vi "主画面.vi"() -> ()   [LabVIEW 2016]
panel:
  out "连接的字符串":string
  in  "邮件按钮":bool
  in  "配置信息":T1={"address"="27.154.58.30", "username"="admin", "password"="std23506", "filename"="一体化微型水质监测站.exe", "localpath"="C:\\Users\\Administrator\\Desktop\\ftp接收文件\\一体化微型水质监测站.exe"}
  out "字符串":string
  in  "启用":bool
  in  "选择站点":bool[](array[boolean])
  out "information":T2(array[cluster])
  in  "多列列表框":i32[](listbox)
  out "子字符串;substring":string
  in  "Port":u16=10000
  in  "empty":refnum<k5>[](array[refnum])
  out "# of Connections":i32
  in  "stop":bool
  in  "listen halted":bool
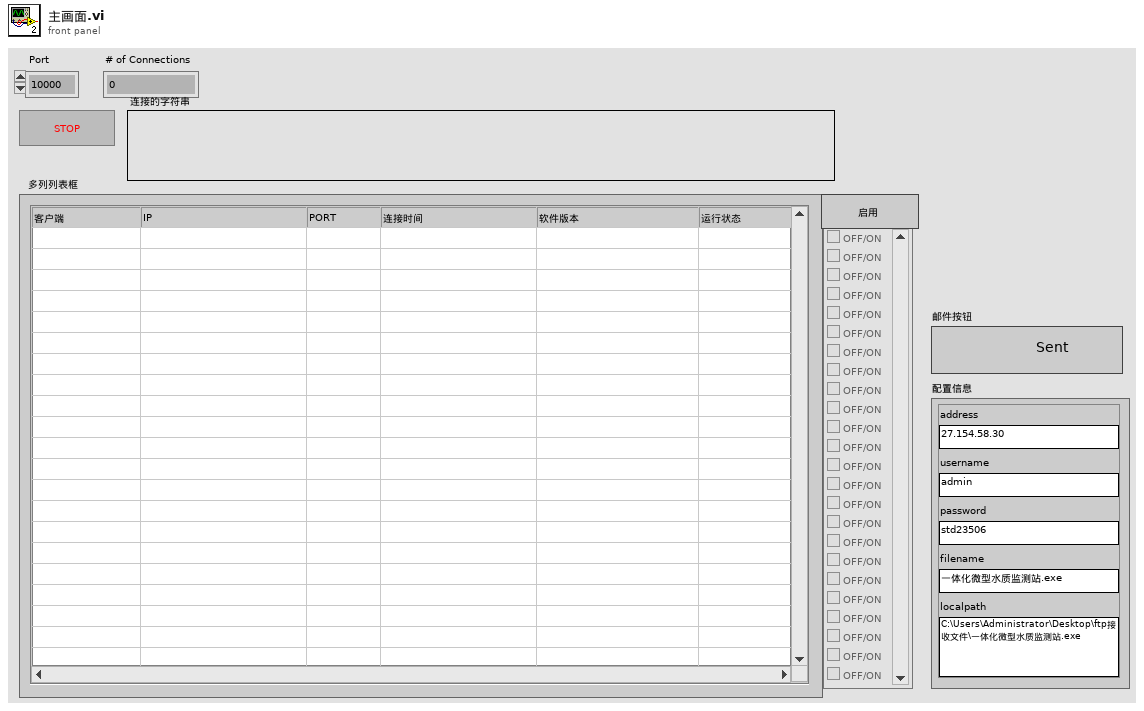
[diagram p1: front panel]
types:
  T1 = cluster{"address":string, "username":string, "password":string, "filename":string, "localpath":string}
  T2 = cluster{"连接ID":refnum<k5>, "名称":string, "远程端口":u16, "连接时间":string}[]
  T3 = enum8{"Enabled", "Disabled", "Disabled and Grayed Out"}
  T4 = enum16{"Standard", "Buffered", "CRLF", "Immediate"}
  T5 = cluster{"远程地址":string[], "远程端口":u16[], "连接ID":refnum<k5>[]}
  T6 = cluster{"连接ID":refnum<k5>, "名称":string, "远程端口":u16, "连接时间":string}
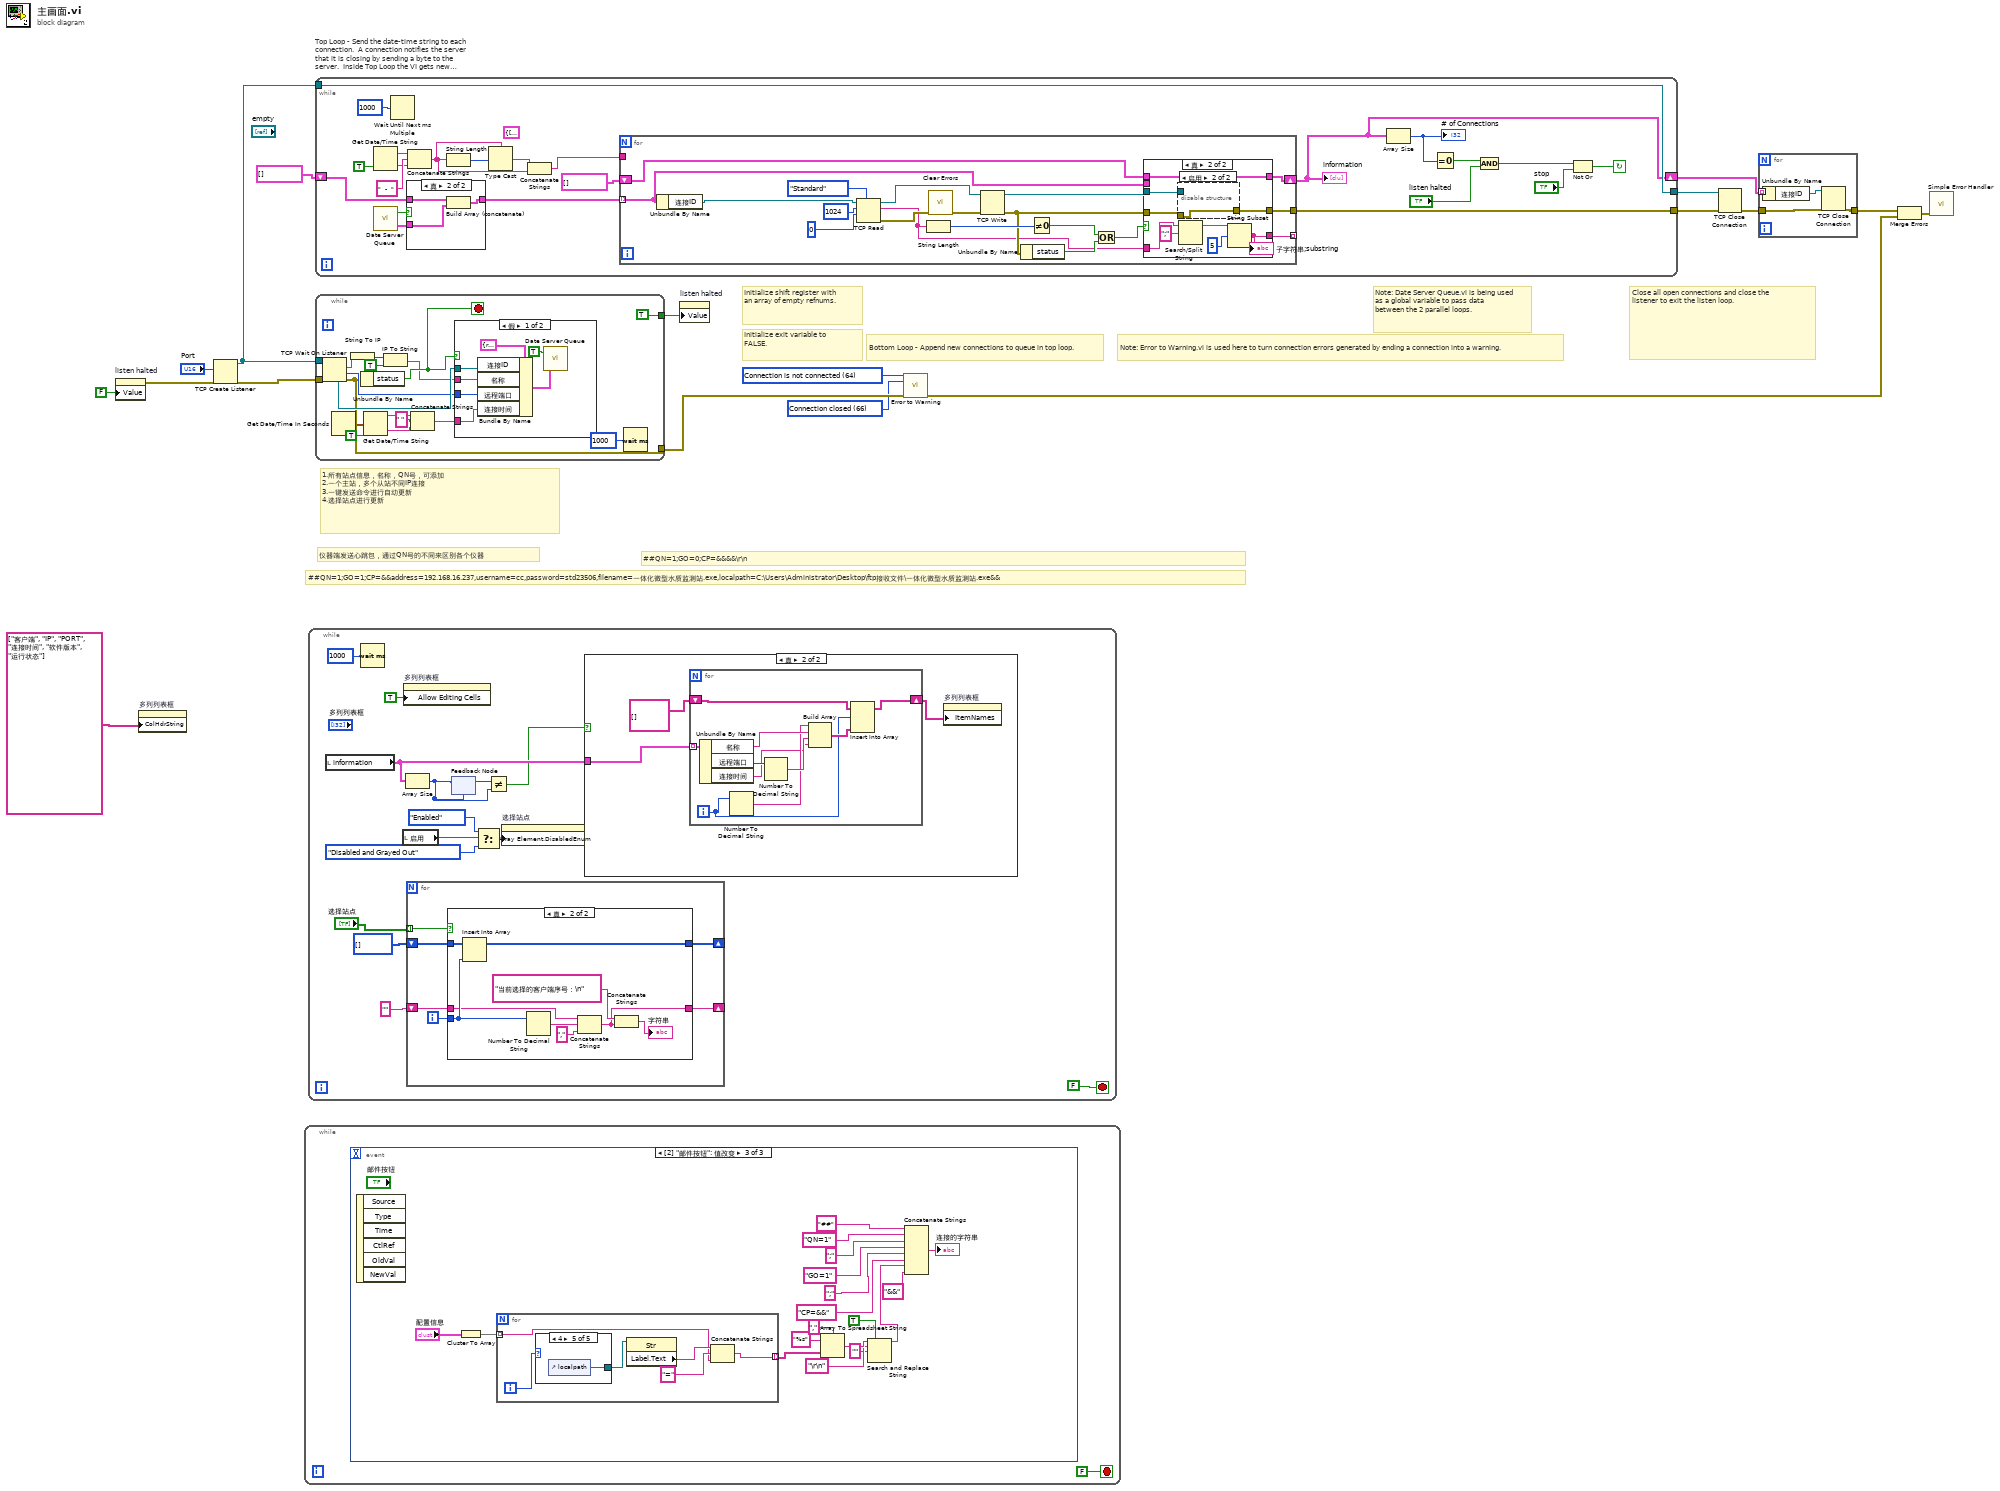
[diagram p0: block diagram]
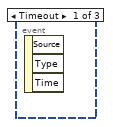
[diagram p2: hidden frame]
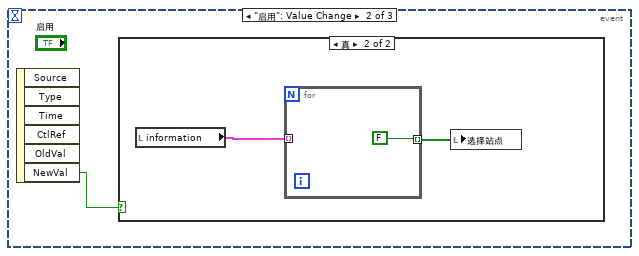
[diagram p3: hidden frame]
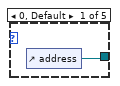
[diagram p5: hidden frame]
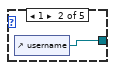
[diagram p6: hidden frame]
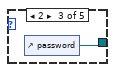
[diagram p7: hidden frame]
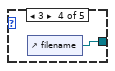
[diagram p8: hidden frame]
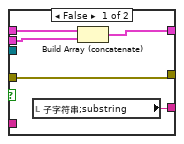
[diagram p11: hidden frame]
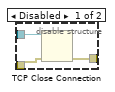
[diagram p12: hidden frame]
diagram:
  w12 = 66 items=["No Error", "Argument Error", "Memory Full", "Out of Zone", "End of File", "File Already Open", "Generic File IO Error", "File Not Found", "File Permission Error", "Disk Full", "Duplicate Path", "Too Many Files Open", "Not Enabled", "Resource File Not Found", "Cannot Add Resource", "Resource Not Found", "Image Not Found", "Image Memory Error", "Pen Does Not Exist", "Config Bad Type", "Config Token Not Found", "Config Parse Error", "Config Memory Error", "Bad External Code Format", "Bad External Code Offset", "External Code Not Present", "Null Window", "Destroy Window Mixup", "Null Menu", "Print Aborted", "Bad Print Record", "Print Driver Error", "Windows Error During Print", "Memory Error During Print", "Print Dialog Error", "Generic Print Error", "Invalid Device Refnum", "Device Not Found", "Device Parameter Error", "Device Unit Error", "Can't Open Device", "Device Call Aborted", "Generic Error", "Cancelled By User", "Object ID Too Low", "Object ID Too High", "Object Not In Heap", "Unknown Heap", "Bad DefProc ID", "DefProc Not In Table", "Message Out Of Range", "Null Method", "Unknown Message", "Manager Call Not Supported", "Bad address", "Connection In progress", "Connection timed out", "Connection is already in progress", "Network attribute not supported", "Network error", "Address in use", "System out of memory", "Connection aborted", "Connection refused", "Connection is not connected", "Connection is already connected", "Connection closed", "Initialize error (interapplication manager)", "Bad occurrence", "Wait on unbound occurrence handler", "Occurrence queue overflow", "Bad path", "Semaphore not signaled", "Unrecognized type (interapplication manager)"] ("2nd Error to Convert")
  w13 = 64 items=["No Error", "Argument Error", "Memory Full", "Out of Zone", "End of File", "File Already Open", "Generic File IO Error", "File Not Found", "File Permission Error", "Disk Full", "Duplicate Path", "Too Many Files Open", "Not Enabled", "Resource File Not Found", "Cannot Add Resource", "Resource Not Found", "Image Not Found", "Image Memory Error", "Pen Does Not Exist", "Config Bad Type", "Config Token Not Found", "Config Parse Error", "Config Memory Error", "Bad External Code Format", "Bad External Code Offset", "External Code Not Present", "Null Window", "Destroy Window Mixup", "Null Menu", "Print Aborted", "Bad Print Record", "Print Driver Error", "Windows Error During Print", "Memory Error During Print", "Print Dialog Error", "Generic Print Error", "Invalid Device Refnum", "Device Not Found", "Device Parameter Error", "Device Unit Error", "Can't Open Device", "Device Call Aborted", "Generic Error", "Cancelled By User", "Object ID Too Low", "Object ID Too High", "Object Not In Heap", "Unknown Heap", "Bad DefProc ID", "DefProc Not In Table", "Message Out Of Range", "Null Method", "Unknown Message", "Manager Call Not Supported", "Bad address", "Connection In progress", "Connection timed out", "Connection is already in progress", "Network attribute not supported", "Network error", "Address in use", "System out of memory", "Connection aborted", "Connection refused", "Connection is not connected", "Connection is already connected", "Connection closed", "Initialize error (interapplication manager)", "Bad occurrence", "Wait on unbound occurrence handler", "Occurrence queue overflow", "Bad path", "Semaphore not signaled", "Unrecognized type (interapplication manager)"] ("1st Error to Convert")
  # "##QN=1;GO=1;CP=&&address=192.168.16.237,username=cc,password=std23506,filename=一体化微型水质监测站.exe,localpath=C:\\Users\\Administrator\\Desktop\\ftp接收文件\\一体化微型水质监测站.exe&&"
  # "##QN=1;GO=0;CP=&&&&\\r\\n"
  # "仪器端发送心跳包，通过QN号的不同来区别各个仪器"
  # "Note: Date Server Queue.vi is being used as a global variable to pass data between the 2 parallel loops."
  # "Note: Error to Warning.vi is used here to turn connection errors generated by ending a connection into a warning."
  # "Initialize shift register with\nan array of empty refnums."
  # "Bottom Loop - Append new connections to queue in top loop."
  # "Initialize exit variable to FALSE."
  # "Close all open connections and close the listener to exit the listen loop."
  # "1.所有站点信息，名称，QN号，可添加\n2.一个主站，多个从站不同IP连接\n3.一键发送命令进行自动更新\n4.选择站点进行更新"
  n1 = property on="listen halted" class="Bool (严格)"("Value"=FALSE) -> (error out=w8:errorcluster)  [unwired: 2 in, 1 out]
  n2 = property on="多列列表框" class="MCListbox (严格)"("ColHdrString"=string[] ["客户端", "IP", "PORT", "连接时间", "软件版本", "运行状态"] ("列首字符串[]")) -> ()  [unwired: 2 in, 2 out]
  n3 = TCP Create Listener(8:w8, 10:"Port") -> (0:w17:errorcluster, 3:w3:refnum<k5>)  [unwired: 4 out]
  n4 = while {
    stop <- FALSE stop-if-true
    n5 = event shown="[2] \"邮件按钮\": 值改变" {
      selector: _ -> [_ _ _]
      dyn-events: _ -> [_ _ _]
      timeout: _ -> [_ _ _]
      event Timeout {
        n6 = event-data() -> ()  [unwired: 1 in, 3 out]
      }
      event "启用": Value Change {
        n7 = event-data() -> ("NewVal"=w20:bool)  [unwired: 1 in, 5 out]
        n8 = case shown="真" w20 {
          frame False {
          }
          frame True {
            n9 = local read "information"() -> (w22:T2)
            n10 = for {
              tunnel: w22 -> [_] mode=indexing
              tunnel: [FALSE] -> w21 mode=indexing
            }
            n11 = local write "选择站点"(w21) -> ()
          }
        }
      }
      event "邮件按钮": Value Change {
        n12 = event-data() -> ()  [unwired: 1 in, 6 out]
        n13 = Cluster To Array(cluster="配置信息") -> (array=w30:string[])
        n14 = for {
          tunnel: w30 -> [w43] mode=indexing
          tunnel: [w42] -> w29 mode=indexing
          i -> [w47]
          n15 = case shown="4" w47 {
            tunnel: [w48 w49 w50 w51 w52] -> w46
            frame 0, Default {
              n16 = control-ref of="address"() -> (w48:refnum<vi>)
            }
            frame 1 {
              n17 = control-ref of="username"() -> (w49:refnum<vi>)
            }
            frame 2 {
              n18 = control-ref of="password"() -> (w50:refnum<vi>)
            }
            frame 3 {
              n19 = control-ref of="filename"() -> (w51:refnum<vi>)
            }
            frame 4 {
              n20 = control-ref of="localpath"() -> (w52:refnum<vi>)
            }
          }
          n21 = property class="Str"(reference=w46) -> ("Label.Text"=w45:string)  [unwired: 1 in, 2 out]
          n22 = Concatenate Strings(w45, "=", w43) -> (w42:string)
        }
        n23 = Array To Spreadsheet String(delimiter (Tab)="," ("分隔符(Tab)"), array=w29, 3:"%s" ("格式字符串")) -> (spreadsheet string=w28:string)
        n24 = Search and Replace String(replace all?=TRUE ("替换全部？(F)"), input string=w28, search string="\r\n" ("搜索字符串"), replace string="" ("替换字符串(\"\")")) -> (result string=w25:string)  [unwired: 4 in, 3 out]
        n25 = Concatenate Strings("##" ("字符串"), "QN=1" ("字符串"), ";" ("字符串"), "GO=1" ("字符串"), ";" ("字符串"), "CP=&&" ("字符串"), w25, "&&" ("字符串")) -> (→"连接的字符串":string)
      }
    }
  }
  n26 = while {
    stop <- FALSE stop-if-true
    n27 = local read "information"() -> (w64:T2)
    n28 = Wait (ms)(milliseconds to wait=u32 1000 ("等待时间（毫秒）")) -> ()  [unwired: 1 out]
    n29 = local read "启用"() -> (w59:bool)
    n30 = property on="多列列表框" class="MCListbox (严格)"("Allow Editing Cells"=TRUE ("允许编辑单元格")) -> ()  [unwired: 2 in, 2 out]
    n31 = Array Size(array=w64) -> (size(s)=w60:i32)
    n32 = for {
      tunnel: "选择站点" -> [w72] mode=indexing
      shift-right: [w69] -> _
      shift-left: i32[] [] -> [w70]
      shift-right: [w67] -> _
      shift-left: "" ("字符串") -> [w68]
      i -> [w71]
      n33 = case shown="真" w72 {
        tunnel: w71 -> [_ w81]
        tunnel: w70 -> [w74 w83]
        tunnel: [w74 w82] -> w69
        tunnel: w68 -> [w73 w79]
        tunnel: [w73 w76] -> w67
        frame False {
        }
        frame True {
          n34 = Insert Into Array(array=w83, new element=w81) -> (w82:i32[])  [unwired: 1 in]
          n35 = Number To Decimal String(number=w81) -> (decimal integer string=w80:string)  [unwired: 1 in]
          n36 = Concatenate Strings(w79, w80, "," ("字符串")) -> (w76:string)
          n37 = Concatenate Strings("当前选择的客户端序号：\n", w76) -> (→"字符串":string)
        }
      }
    }
    n38 = feedback-in #1(w60) -> ()
    n39 = feedback #1(w60) -> (w63:i32)
    n40 = Select(t=T3."Enabled" ("数组元素.禁用"), s=w59, f=T3."Disabled and Grayed Out" ("数组元素.禁用")) -> (s? t:f=w56:T3)
    n41 = Not Equal?(x=w63, y=w60) -> (x != y?=w62:bool)
    n42 = property on="选择站点" class="Arr (严格)"("Array Element.DisabledEnum"=w56) -> ()  [unwired: 2 in, 2 out]
    n43 = case shown="真" w62 {
      tunnel: w64 -> [_ w84]
      frame False {
      }
      frame True {
        n44 = for {
          tunnel: w84 -> [w96] mode=indexing
          shift-right: [w88] -> w85
          shift-left: string[][] [] ("项名") -> [w90]
          i -> [w89]
          n45 = Unbundle By Name(w96) -> ("名称"=w93:string, "远程端口"=w95:u16, "连接时间"=w87:string)
          n46 = Number To Decimal String(number=w89) -> (decimal integer string=w92:string)  [unwired: 1 in]
          n47 = Number To Decimal String(number=w95) -> (decimal integer string=w94:string)  [unwired: 1 in]
          n48 = Build Array(w92, w93, w94, w87) -> (w91:string[])
          n49 = Insert Into Array(array=w90, index (row)=w89, new element=w91) -> (w88:string[][])  [unwired: 1 in]
        }
        n50 = property on="多列列表框" class="MCListbox (严格)"("ItemNames"=w85) -> ()  [unwired: 2 in, 2 out]
      }
    }
  }
  n51 = while "Top Loop - Send the date-time string to each connection.  A connection notifies the server that it is closing by sending a byte to the server.  Inside Top Loop the VI gets new connections one at a time from the queue.  The listen halted control is a hidden control.  It is used to notify the work loop that the listener (bottom loop) has halted.  The top loop will stop if the listener is halted or the stop button is pressed." {
    shift-left: T2 [] -> [w100]
    shift-right: [w97] -> w18
    tunnel: w3 -> [w99]
    tunnel: [w99] -> w16
    tunnel: [w102] -> w7
    stop <- w104 continue-if-true
    (unwired) T5 {"远程地址"=[], "远程端口"=[], "连接ID"=[]}
    n52 = Get Date/Time String(want seconds? (F)=TRUE) -> (date string=w115:string, time string=w108:string)  [unwired: 2 out]
    n53 = call "Date Server Queue.vi"() -> ("值"=w119:T6, "valid?"=w118:bool)  [unwired: 2 in]
    n54 = Wait Until Next ms Multiple(millisecond multiple=u32 1000) -> ()  [unwired: 1 out]
    n55 = case shown="真" w118 {
      tunnel: w119 -> [_ w158]
      tunnel: w100 -> [w157 w160]
      tunnel: [w157 w159] -> w116
      frame False {
      }
      frame True {
        n56 = Build Array (concatenate)(w160, w158) -> (w159:T2)
      }
    }
    n57 = Concatenate Strings(w115, "  -  ", w108) -> (w113:string)
    n58 = String Length(string=w113) -> (length=w114:i32)
    n59 = Type Cast(type=w113, x=w114) -> (*(type *) &x=w112:string)
    n60 = Concatenate Strings(w112, w113) -> (w111:string)
    n61 = for {
      tunnel: w116 -> [w120] mode=indexing
      shift-right: [w138] -> w97
      shift-left: T2 [] -> [w136]
      tunnel: w111 -> [_]
      tunnel: [w137] -> w102
      tunnel: [w122] -> _ mode=indexing
      n62 = Unbundle By Name(w120) -> ("连接ID"=w121:refnum<k5>)
      n63 = TCP Read(connection ID=w121, bytes to read=1024, 7:T4."Standard" ("模式（标准）"), 9:0) -> (connection ID out=w134:refnum<k5>, data out=w123:string, error out=w132:errorcluster)  [unwired: 1 in]
      n64 = String Length(string=w123) -> (length=w131:i32)
      n65 = call <vilib>:"Clear Errors.vi"("error in (no error)"=w132) -> ("error out"=w133:errorcluster)  [unwired: 1 in, 5 out]
      n66 = TCP Write(connection ID=w134, error in (no error)=w133) -> (connection ID out=w125:refnum<k5>, error out=w124:errorcluster)  [unwired: 1 in, 2 out]
      n67 = Unbundle By Name(w124) -> ("status"=w127:bool)
      n68 = Not Equal To 0?(x=w131) -> (x != 0?=w128:bool)
      n69 = Or(x=w128, y=w127) -> (x .or. y?=w126:bool)
      n70 = case shown="真" w126 {
        tunnel: w136 -> [w143 w144]
        tunnel: w125 -> [_ w152]
        tunnel: [w142 w144] -> w138
        tunnel: [w141 w151] -> w137
        tunnel: w124 -> [w141 w150]
        tunnel: w123 -> [_ w146]
        tunnel: [w140 w145] -> w122
        tunnel: w120 -> [w139 _]
        frame False {
          n71 = local read "子字符串;substring"() -> (w140:string)
          n72 = Build Array (concatenate)(w143, w139) -> (w142:T2)
        }
        frame True {
          n73 = disable-structure shown="启用" {
            disable-tunnel: w152 -> [w155 _]
            disable-tunnel: [w154 w156] -> w151
            disable-tunnel: w150 -> [w153 w156]
            frame Disabled {
              n74 = TCP Close Connection(connection ID=w155, error in (no error)=w153) -> (error out=w154:errorcluster)  [unwired: 2 out]
            }
            frame Enabled {
            }
          }
          n75 = Search/Split String(string=w146, search string/char (-)=";" ("搜索字符串/字符(-)")) -> (substring before match=w148:string)  [unwired: 1 in, 2 out]
          n76 = String Subset(string=w148, offset (0)=5 ("偏移量(0)")) -> (substring=w145:string)  [unwired: 1 in]
          "子字符串;substring" <- w145
        }
      }
    }
    "information" <- w97
    n77 = Array Size(array=w97) -> (size(s)=w98:i32)
    "# of Connections" <- w98
    n78 = Equal To 0?(x=w98) -> (x = 0?=w107:bool)
    n79 = And(x=w107, y="listen halted") -> (x .and. y?=w105:bool)
    n80 = Not Or(1:"stop", 2:w105) -> (0:w104:bool)
  }
  n81 = while "Listen loop.  Append new connections to a synchronized queue." {
    tunnel: w3 -> [w177]
    tunnel: w17 -> [w178]
    tunnel: [w167] -> w14
    tunnel: [TRUE] -> w15
    stop <- w173 stop-if-true
    n82 = TCP Wait On Listener(8:w178, 11:w177) -> (0:w167:errorcluster, 1:w168:u16, 2:w172:string, 4:w176:refnum<k5>)  [unwired: 3 out]
    n83 = Get Date/Time In Seconds() -> (seconds since 1Jan1904=w163:timestamp)
    n84 = String To IP(1:w172) -> (0:w171:u32)
    n85 = Unbundle By Name(w167) -> ("status"=w173:bool)
    n86 = Get Date/Time String(seconds (now)=w163, want seconds? (F)=TRUE ("需要秒？(F)")) -> (date string=w164:string, time string=w165:string)  [unwired: 1 in]
    n87 = IP To String(1:TRUE ("句点符号？(F)"), 2:w171) -> (0:w169:string)
    n88 = Concatenate Strings(w164, " " ("字符串"), w165) -> (w162:string)
    n89 = case shown="假" w173 {
      tunnel: w176 -> [w183 _]
      tunnel: w169 -> [w182 _]
      tunnel: w168 -> [w181 _]
      tunnel: w162 -> [w179 _]
      frame False {
        n90 = Bundle By Name(cluster=T6 {"连接ID"=refnum, "名称"="", "远程端口"=0, "连接时间"=""}, "连接ID"=w183, "名称"=w182, "远程端口"=w181, "连接时间"=w179) -> (w184:T6)
        n91 = call "Date Server Queue.vi"("新值"=w184, "set queue? (F: de-queue)"=TRUE) -> ()  [unwired: 2 out]
      }
      frame True {
      }
    }
    n92 = Wait (ms)(milliseconds to wait=u32 1000 ("等待时间（毫秒）")) -> ()  [unwired: 1 out]
  }
  n93 = property on="listen halted" class="Bool (严格)"("Value"=w15) -> ()  [unwired: 2 in, 2 out]
  n94 = call <vilib>:"Error to Warning.vi"("1st Error to Convert"=w13, "2nd Error to Convert"=w12, "error in"=w14) -> ("warning out"=w5:errorcluster)  [unwired: 2 in, 10 out]
  n95 = TCP Close Connection(connection ID=w16, error in (no error)=w7) -> (error out=w6:errorcluster)  [unwired: 2 out]
  n96 = for {
    tunnel: w18 -> [w187] mode=indexing
    tunnel: [w189] -> w11
    tunnel: w6 -> [w188]
    n97 = Unbundle By Name(w187) -> ("连接ID"=w186:refnum<k5>)
    n98 = TCP Close Connection(connection ID=w186, error in (no error)=w188) -> (error out=w189:errorcluster)  [unwired: 2 out]
  }
  n99 = Merge Errors(w11, w5) -> (w10:errorcluster)
  n100 = call <vilib>:"Simple Error Handler.vi"("error in (no error)"=w10) -> ()  [unwired: 1 in, 8 out]
